vi "ROS_Topic_Read_Primative.vi"(0 "ROS in":T1={"topic port"=0, "Node"="", "topic"="", "type"="", "node port"=0, "error "={"status"=FALSE, "code"=0, "source"=""}, "Direction"=enum."Node", "Update (ms)"=1, "queue size"=1}, 1 "Timeout (ms)":i32=500) -> (2 "ROS out":T1={"topic port"=0, "Node"="", "topic"="", "type"="", "node port"=0, "error "={"status"=FALSE, "code"=0, "source"=""}, "Direction"=enum."Node", "Update (ms)"=1, "queue size"=1}, 3 "timed out?":bool, 4 "Reply":string)   [LabVIEW 2012]
doc: "Returns any data received on the topic/service. Only use for subscribers or service clients. Data will need to be parsed."
uses:
  <userlib>/ROSforLV/ROS/Code/SubVIs/_ROSControl.ctl
  <userlib>/ROSforLV/ROS/Code/SubVIs/_ROSDirection.ctl
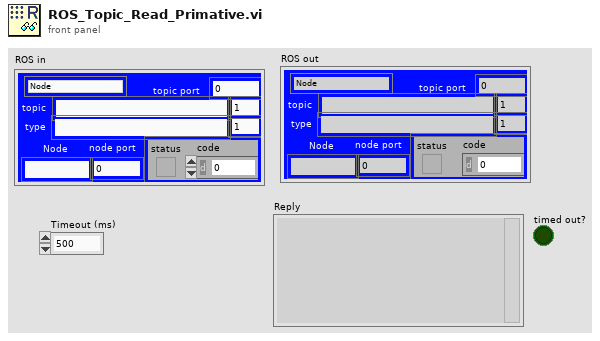
[diagram p1: front panel]
types:
  T1 = typedef "_ROSControl.ctl" = cluster{"topic port":u16, "Node":string, "topic":string, "type":string, "node port":u16, "error ":errorcluster, "Direction":T2, "Update (ms)":u16, "queue size":u16}
  T2 = typedef "_ROSDirection.ctl" = enum16{"Node", "Publisher", "Subscriber", "Service Client"}
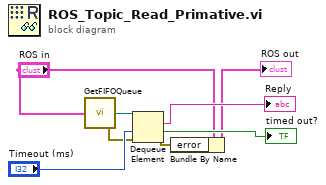
[diagram p0: block diagram]
diagram:
  n1 = call <userlib>:"GetFIFOQueue.vi"("ROS"="ROS in") -> ("error out"=w1:errorcluster, "queue out"=w5:refnum<queue>)  [unwired: 3 in]
  n2 = Dequeue Element(queue=w5, timeout in ms (-1)="Timeout (ms)", error in (no error)=w1) -> (element=→"Reply":string, timed out?=→"timed out?":bool, error out=w3:errorcluster)  [unwired: 1 out]
  n3 = Bundle By Name(cluster="ROS in", "error"=w3) -> (→"ROS out":T1)
